vi "create_data_header_heaz_measurements.vi"() -> (2 "data header":string)   [LabVIEW 2019]
uses:
  Global Variables/global.vi
  Instrument_Setup.vi
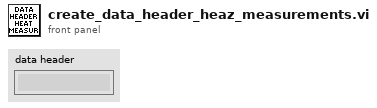
[diagram p1: front panel]
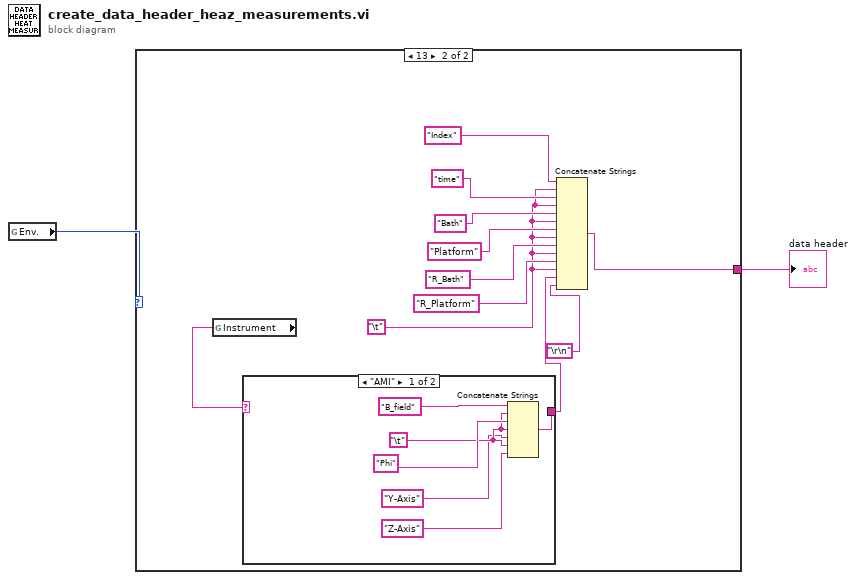
[diagram p0: block diagram]
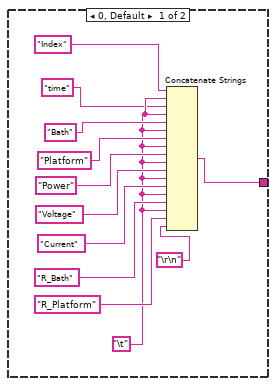
[diagram p2: hidden frame]
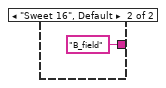
[diagram p3: hidden frame]
diagram:
  n1 = global read "global.vi" "Env."() -> (w1:i32)
  n2 = case shown="13" w1 {
    tunnel: [w6 w21] -> w2
    frame 0, Default {
      w4 = "\t"
      n3 = Concatenate Strings("Index", w4, "time", w4, "Bath", w4, "Platform", w4, "Power", w4, "Voltage", w4, "Current", w4, "R_Bath", w4, "R_Platform", "\r\n") -> (w6:string)
    }
    frame 13 {
      w18 = "\t"
      n4 = global read "Instrument_Setup.vi" "Instrument"() -> (w16:string)
      n5 = case shown="\"AMI\"" w16 {
        tunnel: [w29 "B_field"] -> w15
        frame "AMI" {
          w28 = "\t"
          n6 = Concatenate Strings("B_field", w28, "Phi", w28, "Y-Axis", w28, "Z-Axis") -> (w29:string)
        }
        frame "Sweet 16", Default {
        }
      }
      n7 = Concatenate Strings("Index", w18, "time", w18, "Bath", w18, "Platform", w18, "R_Bath", w18, "R_Platform", w18, w15, "\r\n") -> (w21:string)
    }
  }
  "data header" <- w2
